vi "Check for Single RTL-SDR.vi"(8 "error in (no error)":errorcluster) -> (0 "error out":errorcluster)   [LabVIEW 2017]
doc: "This VI checks if there is one, and only one, RTL-SDR attached."
uses:
  <vilib>/Utility/error.llb/Error Cluster From Error Code.vi
  <vilib>/ErrorRing/Error Ring.xnode
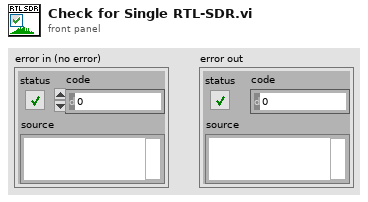
[diagram p1: front panel]
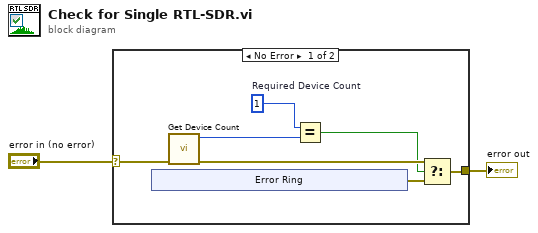
[diagram p0: block diagram]
diagram:
  n1 = case shown="No Error" "error in (no error)" {
    selector: "error in (no error)" -> [w3 w14]
    tunnel: [w8 w14] -> w2
    frame No Error {
      w4 = u32 1  # Required Device Count
      n2 = xnode "Error Ring"() -> ("error out"=w9:errorcluster)
      n3 = call "Get Device Count.vi"("error in (no error)"=w3) -> ("error out"=w7:errorcluster, "Device Count"=w5:u32)  [unwired: 9 in]
      n4 = Equal?(x=w4, y=w5) -> (x = y?=w6:bool)
      n5 = Select(t=w7, s=w6, f=w9) -> (s? t:f=w8:errorcluster)
    }
    frame Error {
    }
  }
  "error out" <- w2
